vi "LabramHR MotorControl.vi"(7 "Control Refnum":refnum<vi>, 8 "error in":errorcluster, 9 "Destination":dbl, 10 "Motor Name":T1=enum."Hole", 11 "Automation Refnum In":refnum<k7>) -> (0 "error out":errorcluster, 2 "MotorID":i32, 3 "Automation Refnum Out":refnum<k7>, 5 "Position":variant)   [LabVIEW 2014]
uses:
  MoveMotor Motor Name.ctl
  MoveMotor Mode.ctl
  GetMotorPosition Mode.ctl
panel:
  in  "stop":bool
  # "LICENSED MATERIALS – PROPERTY OF IBM\nCopyright IBM Corp. 2016,\nALL RIGHTS RESERVED"
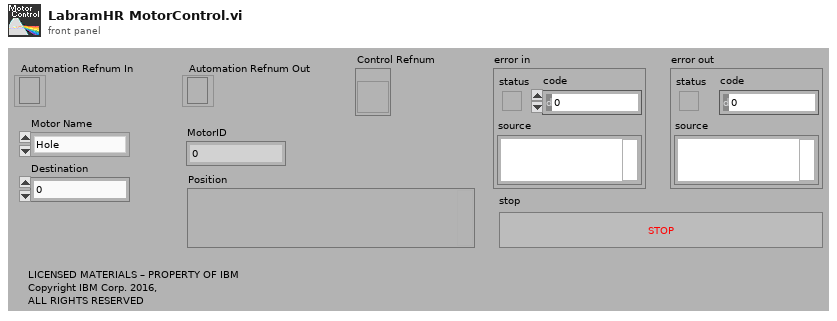
[diagram p1: front panel]
types:
  T1 = typedef "MoveMotor Motor Name.ctl" = enum16{"Spectro", "Premono", "Grating", "Slit", "Hole", "X", "Y", "XT", "YT", "XL", "YL", "Z", "Laser", "Filter", "Objective", "Detector", "Detector Temperature"}
  T2 = typedef "GetMotorPosition Mode.ctl" = u16
  T3 = typedef "MoveMotor Mode.ctl" = u16
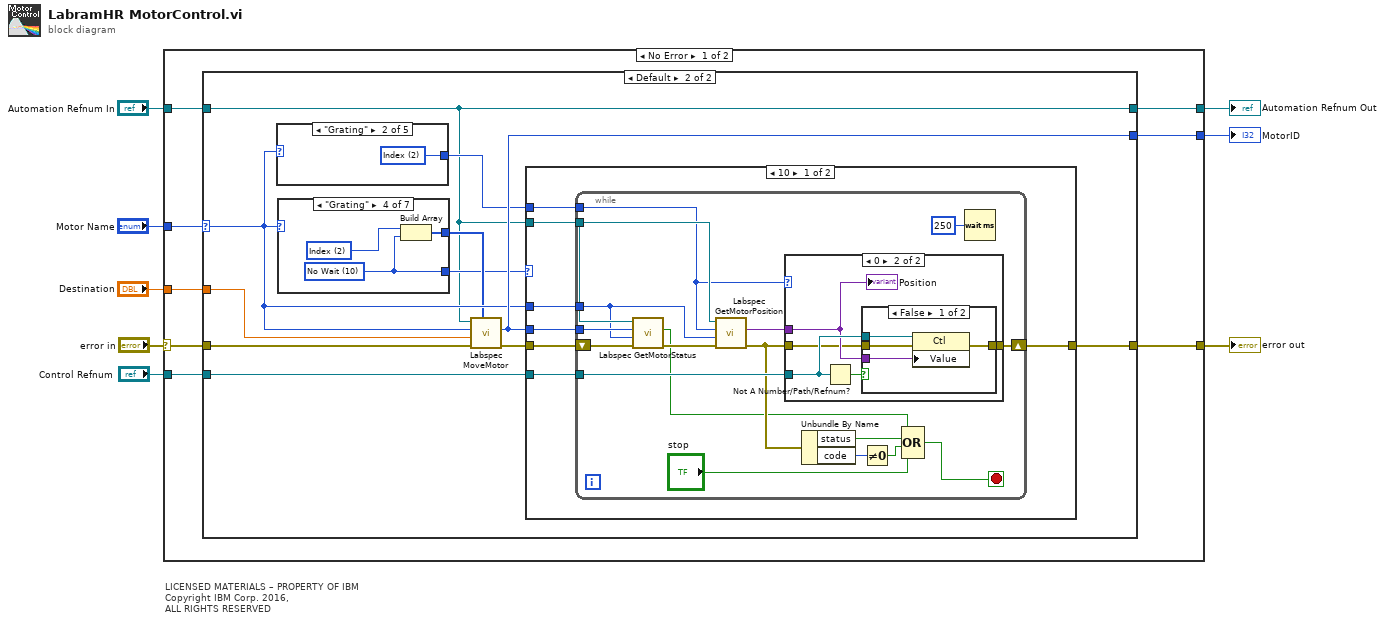
[diagram p0: block diagram]
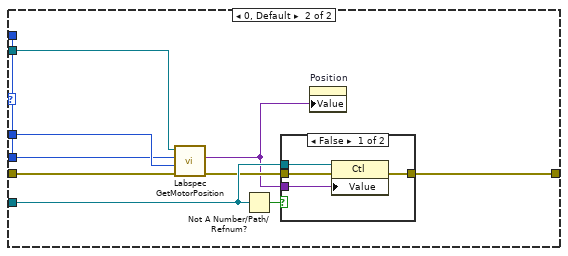
[diagram p5: hidden frame]
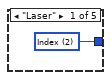
[diagram p7: hidden frame]
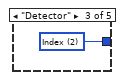
[diagram p8: hidden frame]
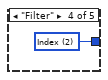
[diagram p9: hidden frame]
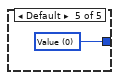
[diagram p10: hidden frame]
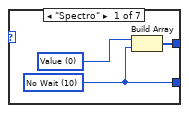
[diagram p11: hidden frame]
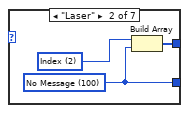
[diagram p12: hidden frame]
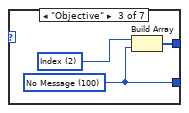
[diagram p13: hidden frame]
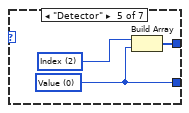
[diagram p14: hidden frame]
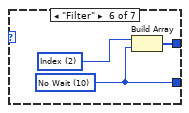
[diagram p15: hidden frame]
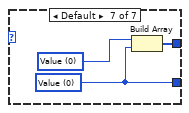
[diagram p16: hidden frame]
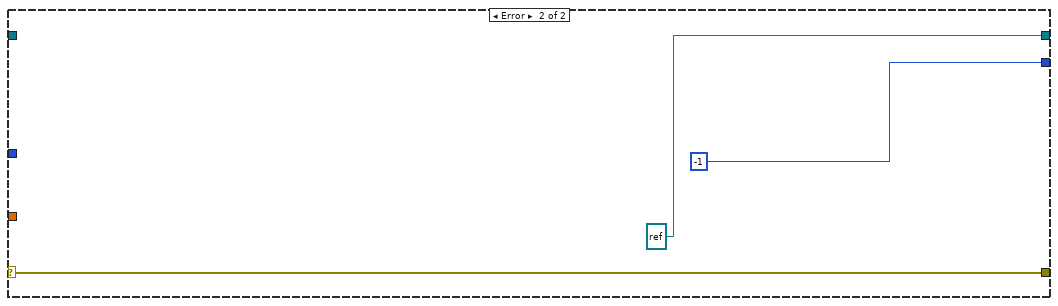
[diagram p17: hidden frame]
diagram:
  # "LICENSED MATERIALS – PROPERTY OF IBM\nCopyright IBM Corp. 2016,\nALL RIGHTS RESERVED"
  n1 = case shown="No Error" "error in" {
    selector: "error in" -> [w11 w107]
    tunnel: "Automation Refnum In" -> [w12 _]
    tunnel: [w9 refnum<k7> refnum ("Automation Refnum")] -> w7
    tunnel: "Destination" -> [w16 _]
    tunnel: "Motor Name" -> [w10 _]
    tunnel: [w13 w107] -> w4
    tunnel: [w15 -1 ("MotorID")] -> w3
    tunnel: "Control Refnum" -> [w14 _]
    frame No Error {
      n2 = case shown="Default" w10 {
        selector: w10 -> [_ w24]
        tunnel: w16 -> [_ w29]
        tunnel: [_ w26] -> w15
        tunnel: w14 -> [_ w28]
        tunnel: [w18 w22] -> w13
        tunnel: w12 -> [w17 w19]
        tunnel: w11 -> [w18 w27]
        tunnel: [w17 w19] -> w9
        frame "Detector Temperature" {
        }
        frame Default {
          n3 = case shown="\"Grating\"" w24 {
            tunnel: [w79 w80 w81 w82 w83] -> w23
            frame "Laser" {
              w79 = T2 2 items=["Value", "Step", "Index", "Size", "Full Size"] ("Mode")
            }
            frame "Grating" {
              w80 = T2 2 items=["Value", "Step", "Index", "Size", "Full Size"] ("Mode")
            }
            frame "Detector" {
              w81 = T2 2 items=["Value", "Step", "Index", "Size", "Full Size"] ("Mode")
            }
            frame "Filter" {
              w82 = T2 2 items=["Value", "Step", "Index", "Size", "Full Size"] ("Mode")
            }
            frame Default {
              w83 = T2 0 items=["Value", "Step", "Index", "Size", "Full Size"] ("Mode")
            }
          }
          n4 = case shown="\"Grating\"" w24 {
            tunnel: [w85 w88 w91 w94 w97 w100 w103] -> w21
            tunnel: [w84 w87 w90 w93 w96 w99 w102] -> w20
            frame "Spectro" {
              w86 = T3 0 items=["Value"=0, "Step"=1, "Index"=2, "String"=3, "Calibrate"=4, "Origin"=5, "Stop"=6, "Value to Step"=7, "No Wait"=10, "No Message"=100] ("Mode")
              w84 = T3 10 items=["Value"=0, "Step"=1, "Index"=2, "String"=3, "Calibrate"=4, "Origin"=5, "Stop"=6, "Value to Step"=7, "No Wait"=10, "No Message"=100] ("Mode")
              n5 = Build Array(w86, w84) -> (w85:T3[])
            }
            frame "Laser" {
              w89 = T3 2 items=["Value"=0, "Step"=1, "Index"=2, "String"=3, "Calibrate"=4, "Origin"=5, "Stop"=6, "Value to Step"=7, "No Wait"=10, "No Message"=100] ("Mode")
              w87 = T3 100 items=["Value"=0, "Step"=1, "Index"=2, "String"=3, "Calibrate"=4, "Origin"=5, "Stop"=6, "Value to Step"=7, "No Wait"=10, "No Message"=100] ("Mode")
              n6 = Build Array(w89, w87) -> (w88:T3[])
            }
            frame "Objective" {
              w92 = T3 2 items=["Value"=0, "Step"=1, "Index"=2, "String"=3, "Calibrate"=4, "Origin"=5, "Stop"=6, "Value to Step"=7, "No Wait"=10, "No Message"=100] ("Mode")
              w90 = T3 100 items=["Value"=0, "Step"=1, "Index"=2, "String"=3, "Calibrate"=4, "Origin"=5, "Stop"=6, "Value to Step"=7, "No Wait"=10, "No Message"=100] ("Mode")
              n7 = Build Array(w92, w90) -> (w91:T3[])
            }
            frame "Grating" {
              w95 = T3 2 items=["Value"=0, "Step"=1, "Index"=2, "String"=3, "Calibrate"=4, "Origin"=5, "Stop"=6, "Value to Step"=7, "No Wait"=10, "No Message"=100] ("Mode")
              w93 = T3 10 items=["Value"=0, "Step"=1, "Index"=2, "String"=3, "Calibrate"=4, "Origin"=5, "Stop"=6, "Value to Step"=7, "No Wait"=10, "No Message"=100] ("Mode")
              n8 = Build Array(w95, w93) -> (w94:T3[])
            }
            frame "Detector" {
              w98 = T3 2 items=["Value"=0, "Step"=1, "Index"=2, "String"=3, "Calibrate"=4, "Origin"=5, "Stop"=6, "Value to Step"=7, "No Wait"=10, "No Message"=100] ("Mode")
              w96 = T3 0 items=["Value"=0, "Step"=1, "Index"=2, "String"=3, "Calibrate"=4, "Origin"=5, "Stop"=6, "Value to Step"=7, "No Wait"=10, "No Message"=100] ("Mode")
              n9 = Build Array(w98, w96) -> (w97:T3[])
            }
            frame "Filter" {
              w101 = T3 2 items=["Value"=0, "Step"=1, "Index"=2, "String"=3, "Calibrate"=4, "Origin"=5, "Stop"=6, "Value to Step"=7, "No Wait"=10, "No Message"=100] ("Mode")
              w99 = T3 10 items=["Value"=0, "Step"=1, "Index"=2, "String"=3, "Calibrate"=4, "Origin"=5, "Stop"=6, "Value to Step"=7, "No Wait"=10, "No Message"=100] ("Mode")
              n10 = Build Array(w101, w99) -> (w100:T3[])
            }
            frame Default {
              w104 = T3 0 items=["Value"=0, "Step"=1, "Index"=2, "String"=3, "Calibrate"=4, "Origin"=5, "Stop"=6, "Value to Step"=7, "No Wait"=10, "No Message"=100] ("Mode")
              w102 = T3 0 items=["Value"=0, "Step"=1, "Index"=2, "String"=3, "Calibrate"=4, "Origin"=5, "Stop"=6, "Value to Step"=7, "No Wait"=10, "No Message"=100] ("Mode")
              n11 = Build Array(w104, w102) -> (w103:T3[])
            }
          }
          n12 = call "Labspec MoveMotor.vi"("Modes"=w21, "error in"=w27, "Position Value"=w29, "Motor Name"=w24, "Automation Refnum In"=w19) -> ("error out"=w25:errorcluster, "MoveID"=w26:i32)  [unwired: 1 in, 4 out]
          n13 = case shown="10" w20 {
            tunnel: w28 -> [w36 w73]
            tunnel: w26 -> [w35 _]
            tunnel: w25 -> [w34 w66]
            tunnel: w19 -> [w33 w72]
            tunnel: w24 -> [w32 w71]
            tunnel: w23 -> [w31 w70]
            tunnel: [w30 w69] -> w22
            frame 10 {
              n14 = while {
                tunnel: w36 -> [w53]
                tunnel: w35 -> [w52]
                tunnel: w33 -> [w50]
                tunnel: w32 -> [w48]
                tunnel: w31 -> [w37]
                shift-right: [w46] -> w30
                shift-left: w34 -> [w51]
                stop <- w40 stop-if-true
                n15 = call "Labspec GetMotorStatus.vi"("error in"=w51, "Motor Name"=w48, "MotorID"=w52, "Automation Refnum In"=w50) -> ("error out"=w49:errorcluster, "Ready?"=w41:bool)  [unwired: 4 in, 1 out]
                n16 = call "Labspec GetMotorPosition.vi"("error in"=w49, "Motor Name"=w48, "Mode"=w37, "Automation Refnum In"=w50) -> ("error out"=w42:errorcluster, "Position"=w47:variant)  [unwired: 1 in, 5 out]
                n17 = case shown="0" w37 {
                  tunnel: w53 -> [_ w59]
                  tunnel: w47 -> [_ w57]
                  tunnel: [w54 w56] -> w46
                  tunnel: w42 -> [w54 w55]
                  frame Default {
                  }
                  frame 0 {
                    n18 = Not A Number/Path/Refnum?(number/path/refnum=w59) -> (NaN/Path/Refnum?=w58:bool)
                    n19 = case shown="False" w58 {
                      tunnel: w59 -> [w63 _]
                      tunnel: w57 -> [w62 _]
                      tunnel: w55 -> [w61 w64]
                      tunnel: [w60 w64] -> w56
                      frame False {
                        n20 = property class="Ctl"(reference=w63, error in=w61, "Value"=w62) -> (error out=w60:errorcluster)  [unwired: 1 out]
                      }
                      frame True {
                      }
                    }
                    "Position" <- w57
                  }
                }
                n21 = Unbundle By Name(w42) -> ("status"=w44:bool, "code"=w45:i32)
                n22 = Not Equal To 0?(x=w45) -> (x != 0?=w43:bool)
                n23 = Compound Arithmetic op=OR(w41, w44, w43, "stop") -> (w40:bool)
                n24 = Wait (ms)(milliseconds to wait=u32 250) -> ()  [unwired: 1 out]
              }
            }
            frame 0, Default {
              n25 = call "Labspec GetMotorPosition.vi"("error in"=w66, "Motor Name"=w71, "Mode"=w70, "Automation Refnum In"=w72) -> ("error out"=w67:errorcluster, "Position"=w65:variant)  [unwired: 1 in, 5 out]
              n26 = Not A Number/Path/Refnum?(number/path/refnum=w73) -> (NaN/Path/Refnum?=w68:bool)
              n27 = case shown="False" w68 {
                tunnel: w73 -> [w77 _]
                tunnel: w65 -> [w76 _]
                tunnel: w67 -> [w75 w78]
                tunnel: [w74 w78] -> w69
                frame False {
                  n28 = property class="Ctl"(reference=w77, error in=w75, "Value"=w76) -> (error out=w74:errorcluster)  [unwired: 1 out]
                }
                frame True {
                }
              }
              n29 = property on="Position" class="LVVar"("Value"=w65) -> ()  [unwired: 2 in, 2 out]
            }
          }
        }
      }
    }
    frame Error {
    }
  }
  "error out" <- w4
  "Automation Refnum Out" <- w7
  "MotorID" <- w3
